vi "Timing.vi"() -> ()   [LabVIEW 2010, in "Twinkle Button.xctl"]
doc: "本VI是为《我和LabVIEW》一书编写的示例。\n关于本书的介绍请参考网页：\nhttp://ruanqizhen.spaces.live.com/blog/cns!5852D4F797C53FB6!4310.entry"
uses:
  Twinkle Button.xctl
  C:/Program Files/National Instruments/LabVIEW 2010/resource/importtools/Common/Event/NISAST Event.lvclass
  Data.ctl
  Message Data.ctl
panel:
  in  "event":refnum<class "NISAST Event.lvclass">
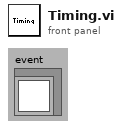
[diagram p1: front panel]
types:
  T1 = typedef "Twinkle Button.xctl/Data.ctl" = enum16{"Red", "Green", "Blue"}
  T2 = typedef "NISAST Event.lvclass/Event Registeration Refnum.ctl" = refnum<event-registration>
  T3 = typedef "Twinkle Button.xctl/Message Data.ctl" = cluster{"cycle":dbl, "led":refnum<vi>, "color":T1}
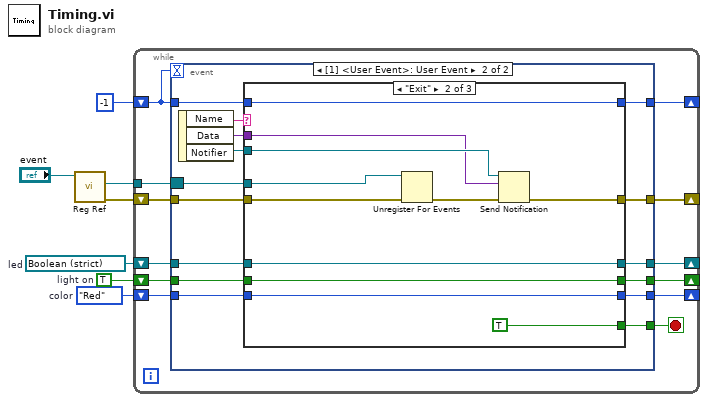
[diagram p0: block diagram]
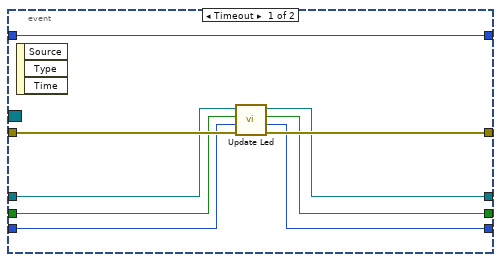
[diagram p2: hidden frame]
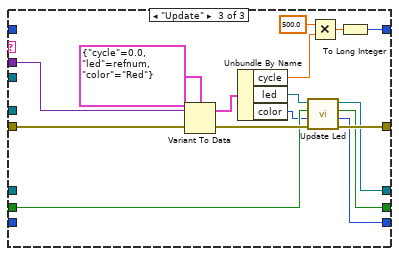
[diagram p4: hidden frame]
diagram:
  w4 = Data."Red"  # color
  w5 = refnum<vi> refnum  # led
  w7 = TRUE  # light on
  n1 = call-dynamic "Reg Ref.vi"("Event in"="event") -> ("error out"=w1:errorcluster, "Event Registration Refnum"=w2:T2)  [unwired: 1 in, 8 out]
  n2 = while {
    tunnel: w2 -> [w19]
    shift-right: [w17] -> _
    shift-left: w1 -> [w18]
    shift-right: [w10] -> _
    shift-left: w7 -> [w11]
    shift-right: [w14] -> _
    shift-left: -1 -> [w15]
    shift-right: [w13] -> _
    shift-left: w5 -> [w9]
    shift-right: [w12] -> _
    shift-left: w4 -> [w8]
    stop <- w16 stop-if-true
    n3 = event shown="[1] <User Event>: User Event" {
      selector: w19 -> [_ w29]
      dyn-events: _ -> [_ _]
      timeout: w15 -> [_ _]
      tunnel: w18 -> [w27 w42]
      tunnel: [w26 w41] -> w17
      tunnel: [_ w39] -> w16
      tunnel: [w28 w37] -> w14
      tunnel: w15 -> [w28 w38]
      tunnel: [w25 w36] -> w13
      tunnel: [w20 w35] -> w12
      tunnel: w11 -> [w23 w34]
      tunnel: [w21 w33] -> w10
      tunnel: w9 -> [w24 w32]
      tunnel: w8 -> [w22 w31]
      event Timeout {
        n4 = event-data() -> ()  [unwired: 4 out]
        n5 = call "Update Led.vi"("error in"=w27, "color"=w22, "light on"=w23, "led"=w24) -> ("error out"=w26:errorcluster, "color"=w20:T1, "light on out"=w21:bool, "led out"=w25:refnum<vi>)  [unwired: 2 in, 2 out]
      }
      event User Event {
        n6 = event-data() -> ("Name"=w43:string, "Data"=w40:variant, "Notifier"=w30:refnum<notifier>)  [unwired: 1 out]
        n7 = case shown="\"Exit\"" w43 {
          tunnel: w42 -> [w44 w53 w73]
          tunnel: [w44 w52 w68] -> w41
          tunnel: w40 -> [_ w50 w75]
          tunnel: [_ TRUE _] -> w39
          tunnel: w38 -> [w48 w58 _]
          tunnel: [w48 w58 w71] -> w37
          tunnel: [w47 w57 w63] -> w36
          tunnel: [w46 w55 w62] -> w35
          tunnel: [w45 w56 w65] -> w33
          tunnel: w34 -> [w45 w56 w66]
          tunnel: w32 -> [w47 w57 _]
          tunnel: w31 -> [w46 w55 _]
          tunnel: w30 -> [_ w51 _]
          tunnel: w29 -> [_ w49 _]
          frame Default {
          }
          frame "Exit" {
            n8 = Unregister For Events(event registration refnum=w49, error in=w53) -> (error out=w54:errorcluster)
            n9 = Send Notification(notification=w50, notifier=w51, error in (no error)=w54) -> (error out=w52:errorcluster)  [unwired: 1 out]
          }
          frame "Update" {
            n10 = Variant To Data(error in=w73, Variant=w75, type=T3 {"cycle"=0.0, "led"=refnum, "color"=enum."Red"} ("data")) -> (error out=w69:errorcluster, data=w72:T3)
            n11 = Unbundle By Name(w72) -> ("cycle"=w61:dbl, "led"=w67:refnum<vi>, "color"=w64:T1)
            n12 = call "Update Led.vi"("error in"=w69, "color"=w64, "light on"=w66, "led"=w67) -> ("error out"=w68:errorcluster, "color"=w62:T1, "light on out"=w65:bool, "led out"=w63:refnum<vi>)  [unwired: 2 in, 2 out]
            n13 = Multiply(x=500.0 ("y"), y=w61) -> (x*y=w70:dbl)
            n14 = To Long Integer(number=w70) -> (32bit integer=w71:i32)
          }
        }
      }
    }
  }
